vi "read txt.vi"() -> ()   [LabVIEW 2012, in "Sendmail.lvrbt"]
uses:
  Sendmail.lvrbt
panel:
  out "String":string
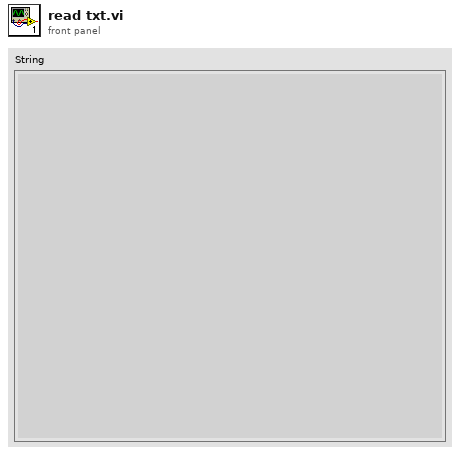
[diagram p1: front panel]
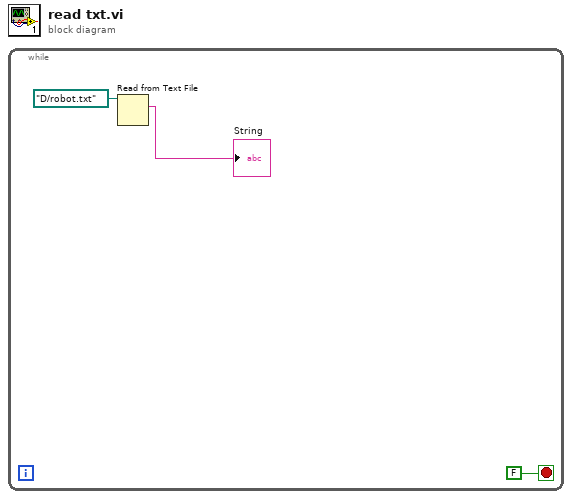
[diagram p0: block diagram]
diagram:
  n1 = while {
    stop <- FALSE stop-if-true
    n2 = Read from Text File(file (use dialog)=path "D:/robot.txt") -> (text=→"String":string)  [unwired: 3 in, 3 out]
  }
